vi "tm410_snap.vi"() -> ()   [LabVIEW 2019]
panel:
  out "Image":u16[][](graph)
  out "Error Out":errorcluster
  # "This is just a simple example of how to capture one image from start to finish."
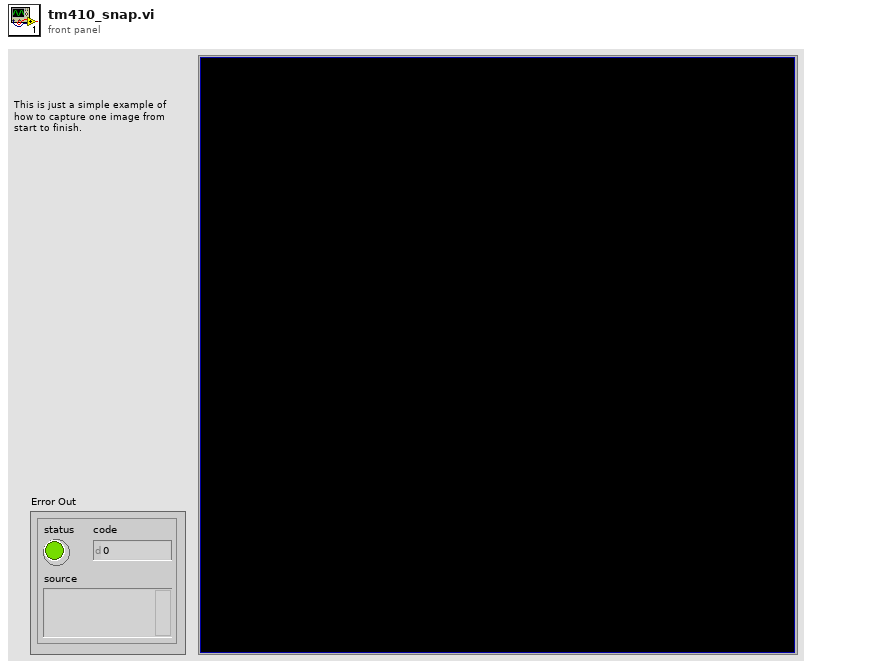
[diagram p1: front panel]
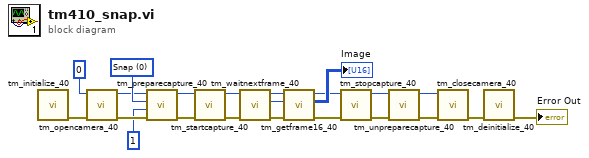
[diagram p0: block diagram]
diagram:
  w14 = 0 items=["Snap", "Sequence"] ("Capture mode")
  n1 = call <userlib>:"tm_initialize_40.vi"() -> ("error out"=w21:errorcluster)  [unwired: 8 in, 3 out]
  n2 = call <userlib>:"tm_opencamera_40.vi"("error in (no error)"=w21, "Camera Index"=u32 0) -> ("error out"=w10:errorcluster, "Handle out"=w11:u32)  [unwired: 7 in, 1 out]
  n3 = call <userlib>:"tm_preparecapture_40.vi"("error in (no error)"=w10, "Frames"=1, "Capture mode"=w14, "Handle in"=w11) -> ("error out"=w12:errorcluster, "Handle out"=w13:u32)  [unwired: 4 in, 2 out]
  n4 = call <userlib>:"tm_startcapture_40.vi"("error in (no error)"=w12, "Handle in"=w13) -> ("error out"=w7:errorcluster, "Handle out"=w6:u32)  [unwired: 8 in]
  n5 = call <userlib>:"tm_waitnextframe_40.vi"("error in (no error)"=w7, "Handle in"=w6) -> ("error out"=w5:errorcluster, "Frame Index"=w1:i32, "Handle out"=w4:u32)  [unwired: 6 in, 1 out]
  n6 = call <userlib>:"tm_getframe16_40.vi"("error in (no error)"=w5, "Frame Index"=w1, "Handle in"=w4) -> ("error out"=w2:errorcluster, "Data"=→"Image":u16[][], "Handle out"=w3:u32)  [unwired: 5 in, 1 out]
  n7 = call <userlib>:"tm_stopcapture_40.vi"("error in (no error)"=w2, "Handle in"=w3) -> ("error out"=w15:errorcluster, "Handle out"=w16:u32)  [unwired: 8 in]
  n8 = call <userlib>:"tm_unpreparecapture_40.vi"("error in (no error)"=w15, "Handle in"=w16) -> ("error out"=w18:errorcluster, "Handle out"=w17:u32)  [unwired: 8 in]
  n9 = call <userlib>:"tm_closecamera_40.vi"("error in (no error)"=w18, "Handle in"=w17) -> ("error out"=w19:errorcluster)  [unwired: 9 in]
  n10 = call <userlib>:"tm_deinitialize_40.vi"("error in (no error)"=w19) -> ("error out"=→"Error Out":errorcluster)  [unwired: 10 in]
